vi "Close Variable Connections.vi"(10 "IO References":T1, 11 "Variable References":T2) -> ()   [LabVIEW 2017]
uses:
  controls/Variable References.ctl
  controls/Control State.ctl
  controls/IO References.ctl
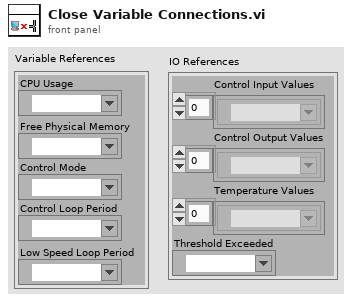
[diagram p1: front panel]
types:
  T1 = typedef "IO References.ctl" = cluster{"Control Input Values":refnum<k21>[], "Control Output Values":refnum<k21>[], "Temperature Values":refnum<k21>[], "Threshold Exceeded":refnum<k21>}
  T2 = typedef "Variable References.ctl" = cluster{"CPU Usage":refnum<k21>, "Free Physical Memory":refnum<k21>, "Control Mode":refnum<k21>, "Control Loop Period":refnum<k21>, "Low Speed Loop Period":refnum<k21>}
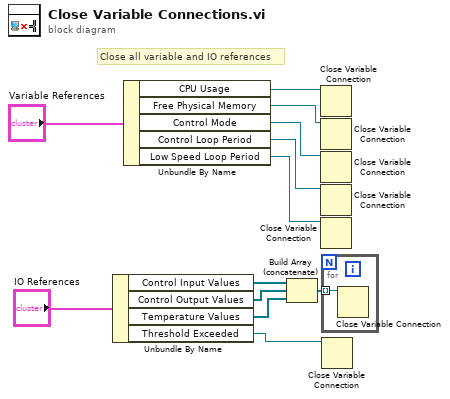
[diagram p0: block diagram]
diagram:
  # "Close all variable and IO references"
  n1 = Unbundle By Name("IO References") -> ("Control Input Values"=w4:refnum<k21>[], "Control Output Values"=w3:refnum<k21>[], "Temperature Values"=w2:refnum<k21>[], "Threshold Exceeded"=w5:refnum<k21>)
  n2 = Unbundle By Name("Variable References") -> ("CPU Usage"=w9:refnum<k21>, "Free Physical Memory"=w10:refnum<k21>, "Control Mode"=w11:refnum<k21>, "Control Loop Period"=w12:refnum<k21>, "Low Speed Loop Period"=w7:refnum<k21>)
  n3 = Build Array (concatenate)(w4, w3, w2) -> (w1:refnum<k21>[])
  n4 = Close Variable Connection(11:w9) -> ()  [unwired: 1 in, 1 out]
  n5 = Close Variable Connection(11:w10) -> ()  [unwired: 1 in, 1 out]
  n6 = Close Variable Connection(11:w11) -> ()  [unwired: 1 in, 1 out]
  n7 = Close Variable Connection(11:w12) -> ()  [unwired: 1 in, 1 out]
  n8 = Close Variable Connection(11:w7) -> ()  [unwired: 1 in, 1 out]
  n9 = for {
    tunnel: w1 -> [w13] mode=indexing
    n10 = Close Variable Connection(11:w13) -> ()  [unwired: 1 in, 1 out]
  }
  n11 = Close Variable Connection(11:w5) -> ()  [unwired: 1 in, 1 out]
